vi "flipflip.vi"() -> ()   [LabVIEW 2009]
panel:
  in  "Boolean 2":bool
  in  "Boolean":bool
  out "Boolean 5":bool
  out "Boolean 4":bool
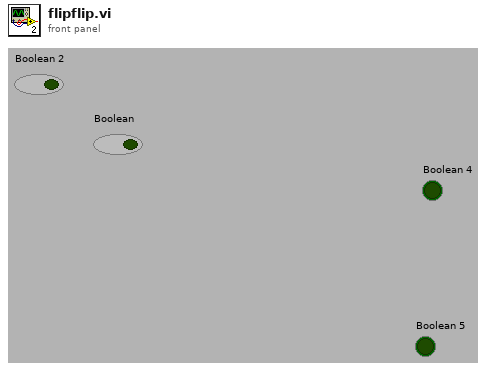
[diagram p1: front panel]
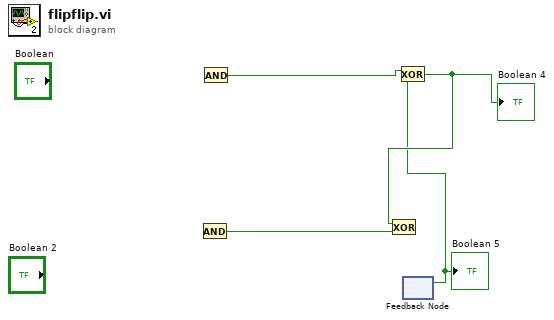
[diagram p0: block diagram]
diagram:
  n1 = And() -> (x .and. y?=w4:bool)  [unwired: 2 in]
  n2 = And() -> (x .and. y?=w5:bool)  [unwired: 2 in]
  n3 = feedback #1() -> (w1:bool)  [unwired: 1 in]
  "Boolean 5" <- w1
  n4 = Exclusive Or(1:w1, 2:w5) -> (0:w3:bool)
  "Boolean 4" <- w3
  n5 = Exclusive Or(1:w4, 2:w3) -> (0:w2:bool)
